vi "appendXMLAcqParam.vi"(8 "Acquisition Parameters":T1, 9 "error in (no error)":errorcluster, 10 "Parent Camera Node":refnum<k20>, 11 "DOM document in":refnum<k20>) -> (0 "error out":errorcluster)   [LabVIEW 2013]
uses:
  <resource>/objmgr/DOMUserDefRef.rc
panel:
  out "White level":dbl
  out "Saturation":dbl
  out "Contrast":dbl
  out "Brightness":dbl
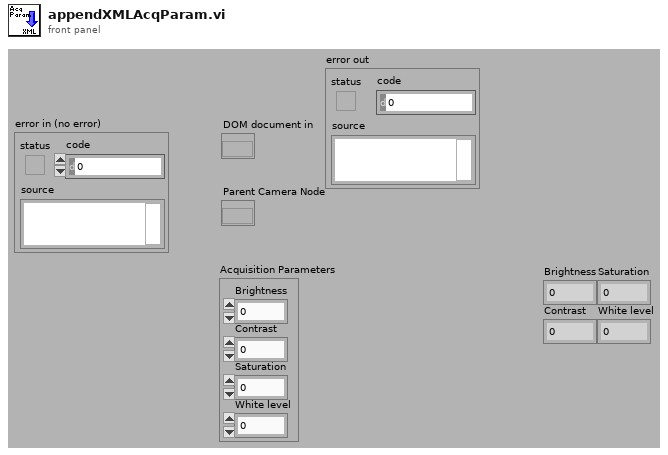
[diagram p1: front panel]
types:
  T1 = cluster{"Brightness":dbl, "Contrast":dbl, "Saturation":dbl, "White level":dbl}
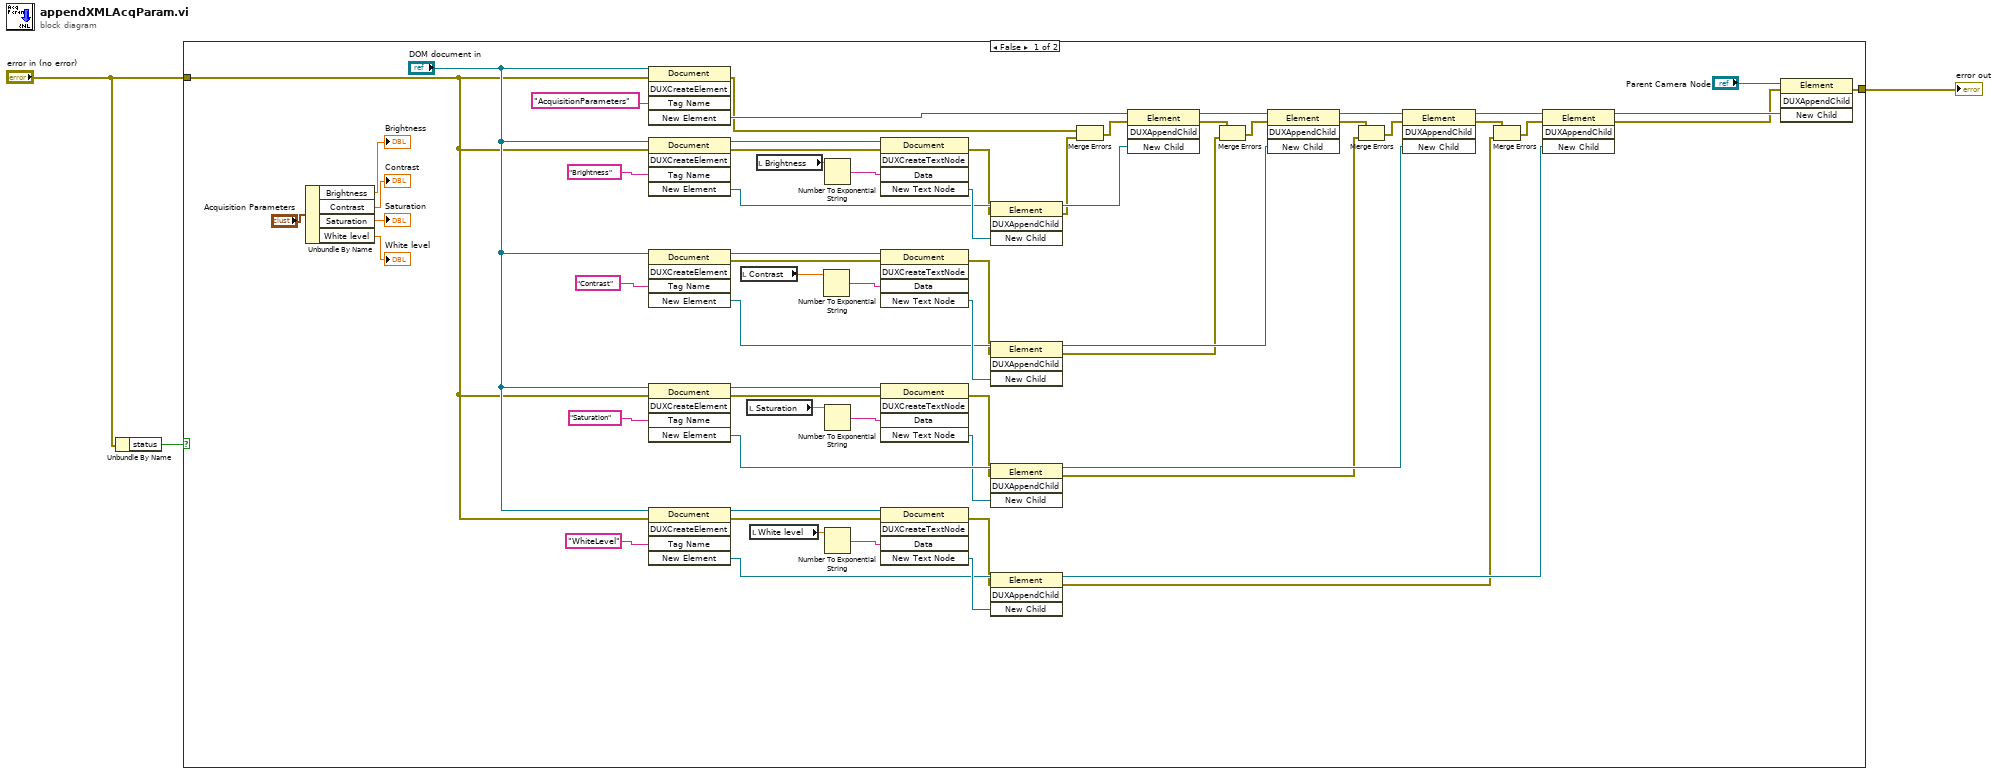
[diagram p0: block diagram]
diagram:
  n1 = Unbundle By Name("error in (no error)") -> ("status"=w2:bool)
  n2 = case shown="False" w2 {
    tunnel: "error in (no error)" -> [w27 w68]
    tunnel: [w6 w68] -> w3
    frame False {
      n3 = Unbundle By Name("Acquisition Parameters") -> ("Brightness"=→"Brightness":dbl, "Contrast"=→"Contrast":dbl, "Saturation"=→"Saturation":dbl, "White level"=→"White level":dbl)
      n4 = invoke class="Document" method="DUXCreateElement"(reference="DOM document in", error in=w27, "Tag Name"="AcquisitionParameters") -> (error out=w17:errorcluster, "New Element"=w62:refnum<k20>)  [unwired: 2 in, 3 out]
      n5 = invoke class="Document" method="DUXCreateElement"(reference="DOM document in", error in=w27, "Tag Name"="Brightness") -> (reference out=w61:refnum<k20>, error out=w26:errorcluster, "New Element"=w57:refnum<k20>)  [unwired: 2 in, 2 out]
      n6 = invoke class="Document" method="DUXCreateElement"(reference="DOM document in", "Tag Name"="Contrast") -> (reference out=w64:refnum<k20>, error out=w25:errorcluster, "New Element"=w59:refnum<k20>)  [unwired: 3 in, 2 out]
      n7 = invoke class="Document" method="DUXCreateElement"(reference="DOM document in", error in=w27, "Tag Name"="Saturation") -> (reference out=w51:refnum<k20>, error out=w24:errorcluster, "New Element"=w53:refnum<k20>)  [unwired: 2 in, 2 out]
      n8 = invoke class="Document" method="DUXCreateElement"(reference="DOM document in", error in=w27, "Tag Name"="WhiteLevel") -> (reference out=w48:refnum<k20>, error out=w23:errorcluster, "New Element"=w46:refnum<k20>)  [unwired: 2 in, 2 out]
      n9 = local read "Contrast"() -> (w33:dbl)
      n10 = local read "Saturation"() -> (w31:dbl)
      n11 = local read "White level"() -> (w28:dbl)
      n12 = local read "Brightness"() -> (w35:dbl)
      n13 = Number To Exponential String(number=w33) -> (E-format string=w32:string)  [unwired: 3 in]
      n14 = Number To Exponential String(number=w35) -> (E-format string=w34:string)  [unwired: 3 in]
      n15 = Number To Exponential String(number=w31) -> (E-format string=w30:string)  [unwired: 3 in]
      n16 = Number To Exponential String(number=w28) -> (E-format string=w29:string)  [unwired: 3 in]
      n17 = invoke class="Document" method="DUXCreateTextNode"(reference=w61, error in=w26, "Data"=w34) -> (error out=w22:errorcluster, "New Text Node"=w58:refnum<k20>)  [unwired: 2 in, 3 out]
      n18 = invoke class="Document" method="DUXCreateTextNode"(reference=w64, error in=w25, "Data"=w32) -> (error out=w21:errorcluster, "New Text Node"=w60:refnum<k20>)  [unwired: 2 in, 3 out]
      n19 = invoke class="Document" method="DUXCreateTextNode"(reference=w51, error in=w24, "Data"=w30) -> (error out=w20:errorcluster, "New Text Node"=w52:refnum<k20>)  [unwired: 2 in, 3 out]
      n20 = invoke class="Document" method="DUXCreateTextNode"(reference=w48, error in=w23, "Data"=w29) -> (error out=w19:errorcluster, "New Text Node"=w47:refnum<k20>)  [unwired: 2 in, 3 out]
      n21 = invoke class="Element" method="DUXAppendChild"(reference=w57, error in=w22, "New Child"=w58) -> (reference out=w56:refnum<k20>, error out=w18:errorcluster)  [unwired: 1 in, 2 out]
      n22 = invoke class="Element" method="DUXAppendChild"(reference=w59, error in=w21, "New Child"=w60) -> (reference out=w55:refnum<k20>, error out=w13:errorcluster)  [unwired: 1 in, 2 out]
      n23 = invoke class="Element" method="DUXAppendChild"(reference=w53, error in=w20, "New Child"=w52) -> (reference out=w43:refnum<k20>, error out=w10:errorcluster)  [unwired: 1 in, 2 out]
      n24 = invoke class="Element" method="DUXAppendChild"(reference=w46, error in=w19, "New Child"=w47) -> (reference out=w42:refnum<k20>, error out=w7:errorcluster)  [unwired: 1 in, 2 out]
      n25 = Merge Errors(w17, w18) -> (w16:errorcluster)
      n26 = invoke class="Element" method="DUXAppendChild"(reference=w62, error in=w16, "New Child"=w56) -> (reference out=w63:refnum<k20>, error out=w14:errorcluster)  [unwired: 1 in, 2 out]
      n27 = Merge Errors(w14, w13) -> (w15:errorcluster)
      n28 = invoke class="Element" method="DUXAppendChild"(reference=w63, error in=w15, "New Child"=w55) -> (reference out=w45:refnum<k20>, error out=w11:errorcluster)  [unwired: 1 in, 2 out]
      n29 = Merge Errors(w11, w10) -> (w12:errorcluster)
      n30 = invoke class="Element" method="DUXAppendChild"(reference=w45, error in=w12, "New Child"=w43) -> (reference out=w44:refnum<k20>, error out=w8:errorcluster)  [unwired: 1 in, 2 out]
      n31 = Merge Errors(w8, w7) -> (w9:errorcluster)
      n32 = invoke class="Element" method="DUXAppendChild"(reference=w44, error in=w9, "New Child"=w42) -> (reference out=w5:refnum<k20>, error out=w4:errorcluster)  [unwired: 1 in, 2 out]
      n33 = invoke class="Element" method="DUXAppendChild"(reference="Parent Camera Node", error in=w4, "New Child"=w5) -> (error out=w6:errorcluster)  [unwired: 1 in, 3 out]
    }
    frame True {
    }
  }
  "error out" <- w3
